vi "Set Tx Generic File Path.vi"(8 "error in":errorcluster, 10 "Frame Array File Path":path, 11 "generic tx section in":T1 format="%.0x") -> (0 "error out":errorcluster, 3 "generic tx section out":T1 format="%.0x")   [LabVIEW 2020, in "AIM ARINC 664 Scripting.lvlib"]
uses:
  <vilib>/NI VeriStand/Custom Device API/Custom Device Item Ref.ctl
  Constants.vi
  AIM ARINC 664 Scripting.lvlib
  <vilib>/NI VeriStand/Custom Device API/Custom Device API.lvlib
  <vilib>/NI VeriStand/Custom Device API/Set Item Property (Dependent File).vi
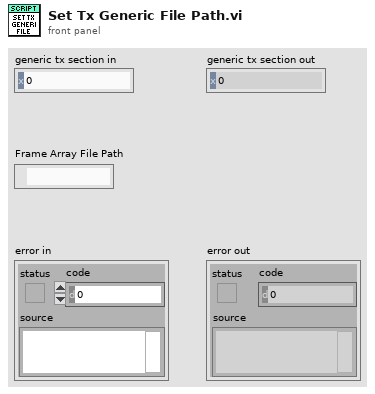
[diagram p1: front panel]
types:
  T1 = typedef "Custom Device API.lvlib/Custom Device Item Ref.ctl" = u64
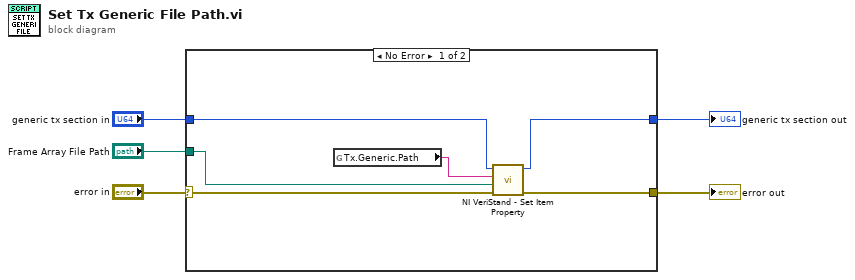
[diagram p0: block diagram]
diagram:
  n1 = case shown="No Error" "error in" {
    selector: "error in" -> [w9 w13]
    tunnel: "generic tx section in" -> [w8 w12]
    tunnel: [w11 w13] -> w4
    tunnel: [w7 w12] -> w3
    tunnel: "Frame Array File Path" -> [w6 _]
    frame No Error {
      n2 = global read "Constants.vi" "Tx.Generic.Path"() -> (w10:string)
      n3 = call-poly <vilib>:"NI VeriStand - Set Item Property.vi"("error in (no error)"=w9, "Path"=w6, "Property Name"=w10, "Item Ref in"=w8) -> ("error out"=w11:errorcluster, "Item Ref out"=w7:T1)  [unwired: 5 in, 1 out]
    }
    frame Error {
    }
  }
  "error out" <- w4
  "generic tx section out" <- w3
